vi "Test.vi"() -> ()   [LabVIEW 2018]
uses:
  Actor/Actor.lvclass
  Actor/Example-Reply.ctl
  Actor/Example-Request.ctl
  Actor/Stop.ctl
  Actor/Actor Class Launched.ctl
  Actor/Event-References.ctl
panel:
  out "Result":T1
  out "Timeout":bool
  out "error out":errorcluster
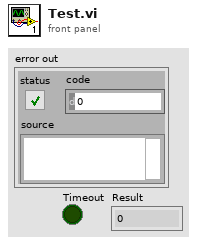
[diagram p1: front panel]
types:
  T1 = typedef "Actor.lvclass/Example-Reply.ctl" = i32
  T2 = cluster{"Example Request-Reply":refnum<event-registration>, "Broadcast":refnum<event-registration>}
  T3 = typedef "Actor.lvclass/Event-References.ctl" = cluster{"Stop":refnum<user-event>, "Launched":refnum<user-event>, "Example-Request":refnum<user-event>}
  T4 = typedef "Actor.lvclass/Example-Request.ctl" = cluster{"Number":bool, "String":string}
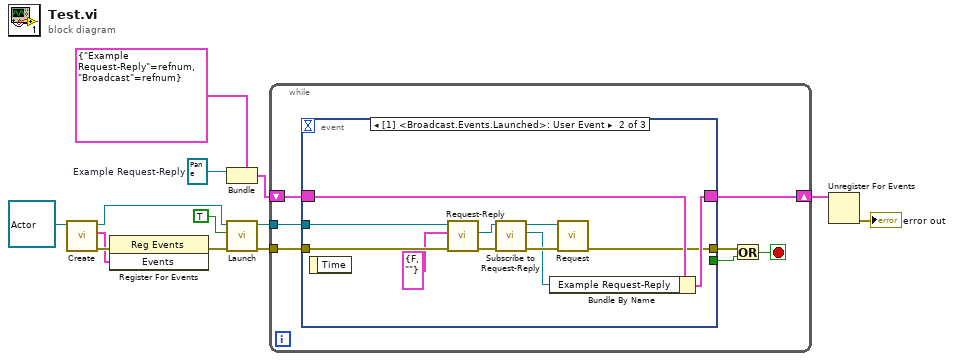
[diagram p0: block diagram]
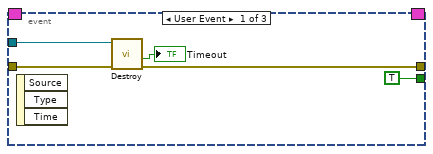
[diagram p2: hidden frame]
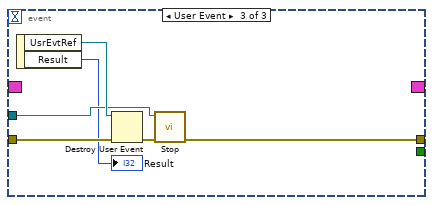
[diagram p3: hidden frame]
diagram:
  w4 = refnum<event-registration> refnum  # Example Request-Reply
  n1 = call "Create.vi"("Actor in"=refnum<class "Actor.lvclass"> refnum) -> ("error out"=w7:errorcluster, "Events"=w6:T3, "API-Reference out"=w1:refnum<k1>)  [unwired: 8 in]
  n2 = register-events(error in=w7, w6) -> (error out=w5:errorcluster)  [unwired: 1 in, 1 out]
  n3 = Bundle(cluster=T2 {"Example Request-Reply"=refnum, "Broadcast"=refnum} ("output cluster"), "Example Request-Reply"=w4) -> (w3:T2)  [unwired: 1 in]
  n4 = call "Launch.vi"("error in (no error)"=w5, "Show Front Panel? (F)"=TRUE, "API-Reference in"=w1) -> ("error out"=w9:errorcluster, "API-Reference out"=w10:refnum<k1>)  [unwired: 6 in, 1 out]
  n5 = while {
    tunnel: w10 -> [w19]
    tunnel: w9 -> [w18]
    shift-right: [w20] -> w11
    shift-left: w3 -> [w17]
    stop <- w14 stop-if-true
    n6 = event shown="[1] <Broadcast.Events.Launched>: User Event" {
      selector: w17 -> [_ w36 _]
      dyn-events: [_ w35 _] -> w20
      timeout: _ -> [_ _ _]
      tunnel: w19 -> [w24 w34 w40]
      tunnel: w18 -> [w23 w33 w41]
      tunnel: [w22 w28 w37] -> w16
      tunnel: [TRUE _ _] -> w15
      event User Event {
        n7 = event-data() -> ()  [unwired: 1 in, 3 out]
        n8 = call "Destroy.vi"("error in (no error)"=w23, "API-Reference in"=w24) -> ("error out"=w22:errorcluster, "Timeout"=→"Timeout":bool)  [unwired: 7 in, 1 out]
      }
      event User Event {
        n9 = event-data() -> ()  [unwired: 1 in, 1 out]
        n10 = call "Request-Reply.vi"("error in (no error)"=w33, "Number"=T4 {"Number"=FALSE, "String"=""}, "API-Reference in"=w34) -> ("error out"=w32:errorcluster, "Example Request Out"=w31:refnum<k1>)  [unwired: 6 in, 1 out]
        n11 = call "Subscribe to Request-Reply.vi"("error in (no error)"=w32, "Example Request in"=w31) -> ("error out"=w30:errorcluster, "Request-Reply Registration"=w27:refnum<event-registration>, "Example Request out"=w29:refnum<k1>)  [unwired: 7 in]
        n12 = Bundle By Name(cluster=w36, "Example Request-Reply"=w27) -> (w35:T2)
        n13 = call "Request.vi"("error in (no error)"=w30, "Example Request in"=w29) -> ("error out"=w28:errorcluster)  [unwired: 9 in]
      }
      event User Event {
        n14 = event-data() -> ("UsrEvtRef"=w42:refnum<user-event>, "Result"=→"Result":T1)  [unwired: 1 in]
        n15 = Destroy User Event(user event=w42, error in=w41) -> (error out=w39:errorcluster)
        n16 = call "Stop.vi"("error in (no error)"=w39, "API-Reference in"=w40) -> ("error out"=w37:errorcluster)  [unwired: 8 in, 1 out]
      }
    }
    n17 = Or(x=w16, y=w15) -> (x .or. y?=w14:bool)
  }
  n18 = Unregister For Events(event registration refnum=w11) -> (error out=→"error out":errorcluster)  [unwired: 1 in]
